vi "Check For Pin Out Of Range.vi"(0 "Arduino Resource":T1={"VISA resource"="", "Board Type"=enum."Arduino Uno", "Connection Type"=enum."USB / Serial", "Bytes Per Packet (15)"=15}, 5 "User Pin Number":u8, 9 "Pin Type":enum16{"Analog", "Digital"}(ring), 11 "error in":errorcluster) -> (4 "Arduino Resource":T1={"VISA resource"="", "Board Type"=enum."Arduino Uno", "Connection Type"=enum."USB / Serial", "Bytes Per Packet (15)"=15}, 15 "error out":errorcluster)   [LabVIEW 2013, in "LabVIEW Interface for Arduino.lvlib"]
uses:
  LabVIEW Interface for Arduino.lvlib
  Private/Type Defs/Arduino Resource.ctl
  Private/Type Defs/Board Type.ctl
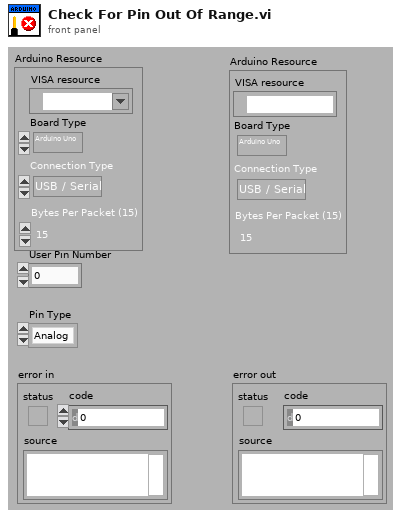
[diagram p1: front panel]
types:
  T1 = typedef "LabVIEW Interface for Arduino.lvlib/Arduino Resource.ctl" = cluster{"VISA resource":refnum<visa-resource-name>, "Board Type":T2, "Connection Type":enum8{"USB / Serial"}, "Bytes Per Packet (15)":u8}
  T2 = typedef "LabVIEW Interface for Arduino.lvlib/Board Type.ctl" = enum16{"Arduino Uno", "Dimuelanove w/Atmega 328", "Mega 2560", "Chipkit Uno32", "Chipkit Max32"}
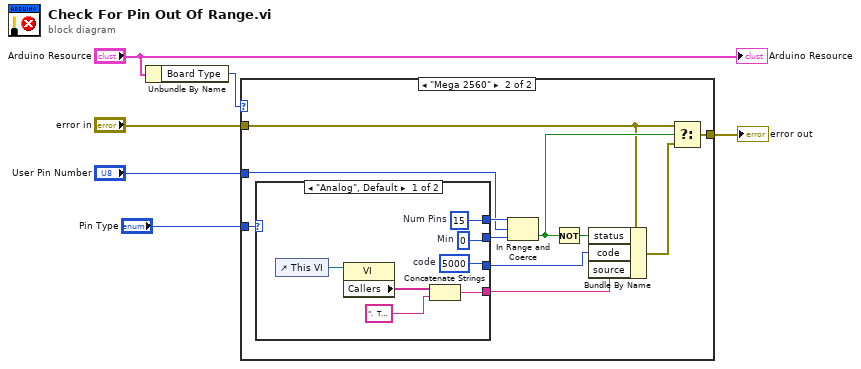
[diagram p0: block diagram]
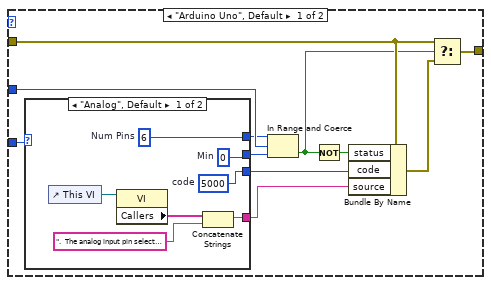
[diagram p2: hidden frame]
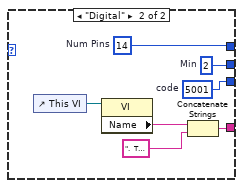
[diagram p3: hidden frame]
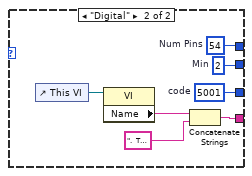
[diagram p4: hidden frame]
diagram:
  n1 = Unbundle By Name("Arduino Resource") -> ("Board Type"=w3:T2)
  n2 = case shown="\"Mega 2560\"" w3 {
    tunnel: "User Pin Number" -> [w16 w35]
    tunnel: "error in" -> [w12 w36]
    tunnel: [w17 w33] -> w5
    tunnel: "Pin Type" -> [w15 w34]
    frame "Arduino Uno", Default {
      n3 = case shown="\"Analog\", Default" w15 {
        tunnel: [w23 w31] -> w14
        tunnel: [w24 w30] -> w13
        tunnel: [w22 w29] -> w8
        tunnel: [w18 w25] -> w7
        frame "Analog", Default {
          w22 = 5000  # code
          w24 = u8 6  # Num Pins
          w23 = u8 0  # Min
          n4 = control-ref of="This VI"() -> (w20:refnum<vi>)
          n5 = property class="VI"(reference=w20) -> ("Callers"=w21:string[])  [unwired: 1 in, 2 out]
          n6 = Concatenate Strings(w21, ".  The analog input pin selected does not exist on the specified board." ("source")) -> (w18:string)
        }
        frame "Digital" {
          w29 = 5001  # code
          w30 = u8 14  # Num Pins
          w31 = u8 2  # Min
          n7 = control-ref of="This VI"() -> (w27:refnum<vi>)
          n8 = property class="VI"(reference=w27) -> ("Name"=w28:string)  [unwired: 1 in, 2 out]
          n9 = Concatenate Strings(w28, ".  The digital pin selected does not exist on the specified board or is in use (pin 0 and 1 are reserved for communication with LabVIEW)." ("source")) -> (w25:string)
        }
      }
      n10 = In Range and Coerce(upper limit=w13, x=w16, lower limit=w14) -> (In Range?=w10:bool)  [unwired: 1 out]
      n11 = Not(x=w10) -> (.not. x?=w11:bool)
      n12 = Bundle By Name(cluster=w12, "status"=w11, "code"=w8, "source"=w7) -> (w9:errorcluster)
      n13 = Select(t=w12, s=w10, f=w9) -> (s? t:f=w17:errorcluster)
    }
    frame "Mega 2560" {
      n14 = case shown="\"Analog\", Default" w34 {
        tunnel: [w48 w56] -> w42
        tunnel: [w49 w55] -> w41
        tunnel: [w43 w50] -> w38
        tunnel: [w47 w54] -> w32
        frame "Analog", Default {
          w47 = 5000  # code
          w49 = u8 15  # Num Pins
          w48 = u8 0  # Min
          n15 = control-ref of="This VI"() -> (w45:refnum<vi>)
          n16 = property class="VI"(reference=w45) -> ("Callers"=w46:string[])  [unwired: 1 in, 2 out]
          n17 = Concatenate Strings(w46, ".  The analog input pin selected does not exist on the specified board." ("source")) -> (w43:string)
        }
        frame "Digital" {
          w54 = 5001  # code
          w55 = u8 54  # Num Pins
          w56 = u8 2  # Min
          n18 = control-ref of="This VI"() -> (w52:refnum<vi>)
          n19 = property class="VI"(reference=w52) -> ("Name"=w53:string)  [unwired: 1 in, 2 out]
          n20 = Concatenate Strings(w53, ".  The digital pin selected does not exist on the specified board or is in use (pin 0 and 1 are reserved for communication with LabVIEW)." ("source")) -> (w50:string)
        }
      }
      n21 = In Range and Coerce(upper limit=w41, x=w35, lower limit=w42) -> (In Range?=w39:bool)  [unwired: 1 out]
      n22 = Not(x=w39) -> (.not. x?=w40:bool)
      n23 = Bundle By Name(cluster=w36, "status"=w40, "code"=w32, "source"=w38) -> (w37:errorcluster)
      n24 = Select(t=w36, s=w39, f=w37) -> (s? t:f=w33:errorcluster)
    }
  }
  "error out" <- w5
  "Arduino Resource" <- "Arduino Resource"
